vi "ROI grp-Rename group.vi"() -> ()   [LabVIEW 2013]
uses:
  Global variables/gl_Functional Imaging-Global variables.vi
  Globals/gl_ROI grp window globals.vi
panel:
  out "error out":errorcluster
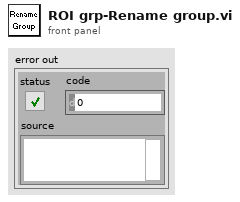
[diagram p1: front panel]
types:
  T1 = typedef "Functional Imging UI Refs.ctl" = cluster{"Menu ref":refnum<k9>, "Image control":refnum<vi>, "VI ref":refnum<vi>, "XGrapher":refnum<vi>, "Smoothing":refnum<vi>, "POI Averaging":refnum<vi>, "Normalize":refnum<vi>, "POI data points in each trial":refnum<vi>, "Channel":refnum<vi>, "Experiment data folder path":refnum<vi>, "[ROI vis]":refnum<vi>, "[Groups] visbl":T2, "Group Name":refnum<vi>, "POI index":refnum<vi>, "Trial No.":refnum<vi>, "Intensity Zoom":refnum<vi>, "Trial Cursor Enabled":refnum<vi>, "Number of Trials (ind 1)":refnum<vi>, "Number of Trials (ind 2)":refnum<vi>, "MiniScans Available":refnum<vi>, "POI Available":refnum<vi>, "Defer graph updates":refnum<vi>, "Waveform selector":refnum<vi>, "#of selected POI":refnum<vi>, "#of selected MiniScans":refnum<vi>, "#of selected groups":refnum<vi>, "Max Z-Projection":refnum<vi>, "Z-Plane Selector":refnum<vi>, "Index of miniscan point to visualise":refnum<vi>, "ROI vis. mode":refnum<vi>, "Total # of points":refnum<vi>, "Index of group clicked on":refnum<vi>, "Pane 1":refnum<vi>, "Pane 2":refnum<vi>, "Pane 3":refnum<vi>, "Pane 4":refnum<vi>, "Pane 5":refnum<vi>, "Pane 6":refnum<vi>, "Deselect all ROI":refnum<vi>, "Deselect all groups":refnum<vi>}
  T2 = typedef "Groups array referecne.ctl" = refnum<vi>
  T3 = typedef "Group sel cluster.ctl" = cluster{"Group number":string, "Group Name":string, "Visibility":bool, "Highlight":bool}
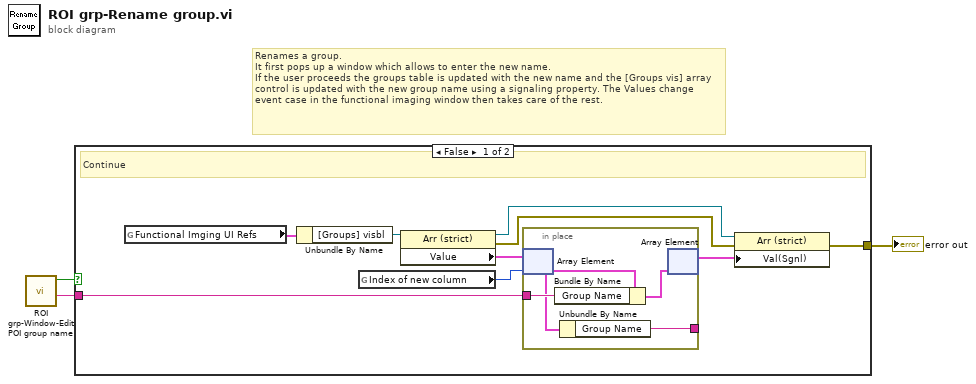
[diagram p0: block diagram]
diagram:
  # "Renames a group.\nIt first pops up a window which allows to enter the new name.\nIf the user proceeds the groups table is updated with the new name and the [Groups vis] array control is updated with the new group name using a signaling property. The Values change event case in the functional imaging window then takes care of the rest."
  n1 = call "ROI grp-Window-Edit POI group name.vi"() -> ("Group Name out"=w2:string, "Cancelled"=w3:bool)  [unwired: 10 in]
  n2 = case shown="False" w3 {
    tunnel: w2 -> [w6 _]
    tunnel: [w4 _] -> w1
    frame False {
      # "Continue"
      n3 = global read "gl_Functional Imaging-Global variables.vi" "Functional Imging UI Refs"() -> (w12:T1)
      n4 = Unbundle By Name(w12) -> ("[Groups] visbl"=w11:T2)
      n5 = global read "gl_ROI grp window globals.vi" "Index of new column"() -> (w5:i32)
      n6 = property on="Property Node" class="Arr (strict)"(reference=w11) -> (reference out=w9:T2, error out=w8:errorcluster, "Value"=w10:T3[])  [unwired: 1 in]
      n7 = in-place {
        in-place-border: w6 -> [w15]
        in-place-border: [w13] -> _
        n8 = in-place-array #1(w10, w5) -> (w14:T3)
        n9 = Bundle By Name(cluster=w14, "Group Name"=w15) -> (w16:T3)
        n10 = Unbundle By Name(w14) -> ("Group Name"=w13:string)
        n11 = in-place-array #1(w16) -> (w7:T3[])  [unwired: 1 out]
      }
      n12 = property on="Property Node" class="Arr (strict)"(reference=w9, error in=w8, "Val(Sgnl)"=w7) -> (error out=w4:errorcluster)  [unwired: 1 out]
    }
    frame True {
      # "Cancelled"
    }
  }
  "error out" <- w1
